vi "PH_Timing.PC link SRDG 645 Channel Infos.vi"(0 "i ref in":refnum<vi>, 1 "data":i8[](array[numeric]), 2 "Service Name":string="N/A", 3 "typeDescriptor":string="D:N", 4 "no link":bool, 5 "error in":errorcluster) -> (14 "i ref out":refnum<vi>, 19 "error out":errorcluster)   [LabVIEW 2014, in "PH_Timing.lvlib"]
doc: "This VI writes the incoming information to own attributes and sets GUI elements."
uses:
  PH_Timing.lvlib
  instr.lib/Stanford Research DG645/Driver/Channel.ctl
  instr.lib/Stanford Research DG645/Stanford Research DG645 - Driver.lvlib
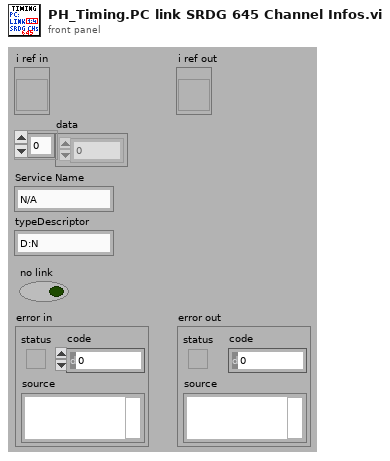
[diagram p1: front panel]
types:
  T1 = typedef "PH_Timing.lvlib/PH_Timing.i attribute.ctl" = cluster{"Sequencer":cluster{"linked?":bool, "Proc State":string, "Ref State":refnum<vi>}, "Gate Generator":cluster{"GD":cluster{"Device Status":T2, "linked?":bool}, "Settings":T3, "GUI Ref":refnum<vi>}, "Interlock Bypass":cluster{"Instancename":string, "Switch linked?":bool, "Device Status":T2, "Ref Status":refnum<vi>}, "Roughtuner":cluster{"Settings":T4, "GUI Ref":refnum<vi>, "GD":cluster{"Device Status":T2, "linked?":bool}}, "0,5Hz Gater":cluster{"Settings":T5, "GUI Ref":refnum<vi>, "GD":cluster{"Device Status":T2, "linked?":bool}}, "Slow Trigger":cluster{"Settings":T6, "GUI Ref":refnum<vi>, "Service ID Delay":i32, "Service ID Ext Trig":i32, "Wanted Settings":T6}, "Timing Mode":cluster{"Mode":T7, "GUI Ref":refnum<vi>, "Service ID T2":i32, "Service ID Mode":i32, "Wanted Mode":T7}, "ns Generator":cluster{"Settings":T8, "ns Generator Settings":refnum<vi>, "GD":cluster{"Device Status":T2, "linked?":bool}}, "Phase FEs":cluster{"Settings":T11, "GUI Ref":refnum<vi>, "Service ID Phase":i32, "Wanted Settings":T11}, "GD GUI Refs":refnum<vi>[], "Heads":T12[], "GUI Ref Delete":refnum<vi>}
  T2 = typedef "PH_StatusHandler.lvlib/PH_StatusHandler.Status.ctl" = i16
  T3 = typedef "PH_Timing.lvlib/PH_Timing.GateGen.ctl" = cluster{"Instance":string, "Channel Gate":i32, "Channel T2":i32, "Width Gate":dbl, "Width T2":dbl, "Delay Gate":dbl, "Delay T2":dbl, "Gate activ":bool, "T2 activ":bool, "System Mode":enum16{"Normal", "Single", "Burst", "Duty Cycle"}}
  T4 = typedef "PH_Timing.lvlib/PH_Timing.Roughtuner.ctl" = cluster{"Instance":string, "Phase PHELIX / UNILAC":cluster{"Channel":u16, "relative to":u16, "Delay [ms]":dbl}, "Pulse Length":cluster{"Channel":u16, "relative to":u16, "Delay [ms]":dbl}, "Trigger":cluster{"externally?":bool, "Rate [Hz]":dbl}}
  T5 = typedef "PH_Timing.lvlib/PH_Timing.0.5HzGater.ctl" = cluster{"Instance":string, "Channel ns FE Delay":i32, "Channel 0.5Hz":i32, "Width ns FE Delay":dbl, "Width 0.5Hz":dbl, "Delay ns FE Delay":dbl, "Delay 0.5Hz":dbl, "ns FE Delay active":bool, "0.5Hz activ":bool, "ns FE Delay inverted":bool, "0.5Hz inverted":bool}
  T6 = typedef "PH_Timing.lvlib/PH_Timing.Slow Trigger Settings.ctl" = cluster{"Delay":dbl, "externally triggered?":bool}
  T7 = typedef "PH_Timing.lvlib/PH_Timing.Timing Mode.ctl" = cluster{"T2":i16, "Modeselector":enum32{"10 Hz", "0.5 Hz", "Shot"}}
  T8 = typedef "PH_Timing.lvlib/PH_Timing.ns Generator.ctl" = cluster{"Instance":string, "Phase fs / ns FE":cluster{"Channel":T9, "Settings":T10}}
  T9 = typedef "Stanford Research DG645 - Driver.lvlib/Channel.ctl" = i32
  T10 = typedef "PH_SRDG645.lvlib/PH_SRDG645.Channel Settings.ctl" = cluster{"Delay [s]":dbl, "relative to":i32}
  T11 = typedef "PH_Timing.lvlib/PH_Timing.Phase FEs.ctl" = cluster{"Phase":dbl}
  T12 = typedef "PH_Timing.lvlib/PH_Timing.PU Data.ctl" = cluster{"linked?":bool, "Data":T13, "GD":cluster{"Device Status":T2, "linked?":bool}, "GUI Ref":refnum<vi>, "PU":T14}
  T13 = typedef "PH_Timing.lvlib/PH_Timing.PU Info.ctl" = cluster{"Act CH?":bool, "GD":string, "CH":i32, "Delay":dbl, "active":bool, "in Use?":bool}
  T14 = typedef "PH_PP_Common.lvlib/PH_PP_Common.PUs.ctl" = enum16{"no Info", "PA-19mm-1", "PA-19mm-2", "PA-45mm-PILC", "PA-45mm-MAIN", "MA-PU-1", "MA-PU-2", "MA-PU-3", "MA-PU-4", "MA-PU-5", "MA-PU-6", "MA-FR", "MA-PILC", "PA-45mm-DP"}
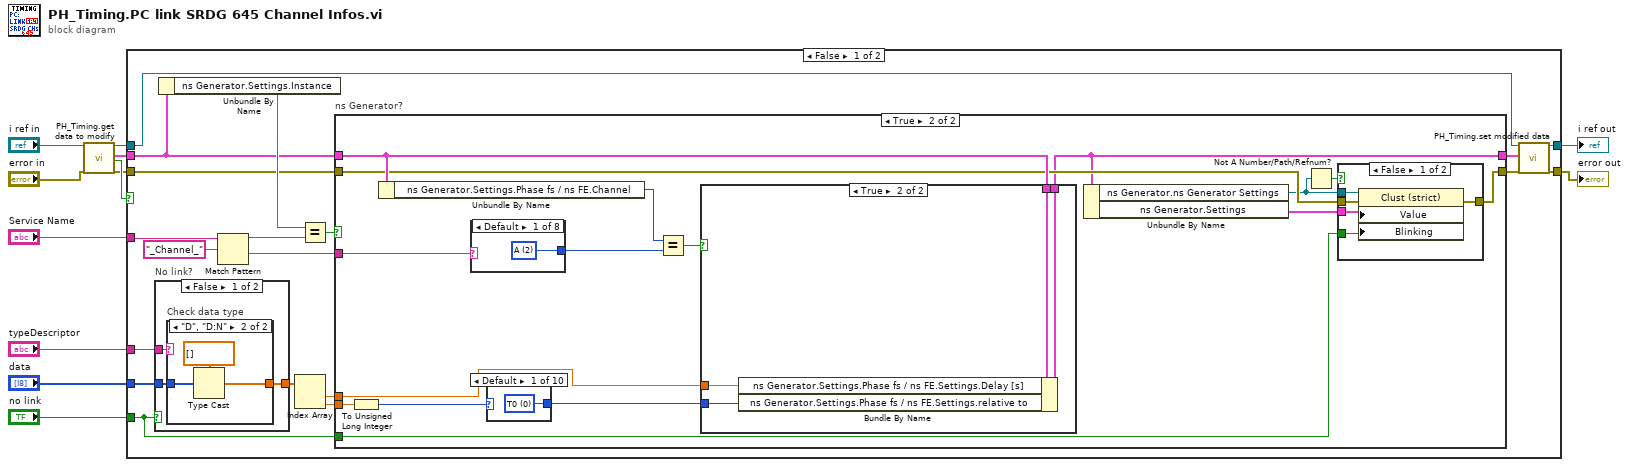
[diagram p0: block diagram]
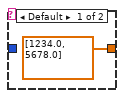
[diagram p2: hidden frame]
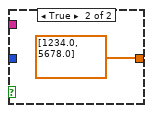
[diagram p3: hidden frame]
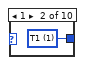
[diagram p5: hidden frame]
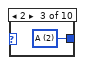
[diagram p6: hidden frame]
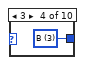
[diagram p7: hidden frame]
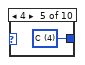
[diagram p8: hidden frame]
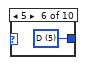
[diagram p9: hidden frame]
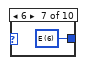
[diagram p10: hidden frame]
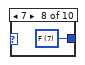
[diagram p11: hidden frame]
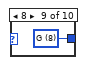
[diagram p12: hidden frame]
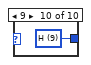
[diagram p13: hidden frame]
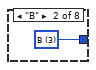
[diagram p15: hidden frame]
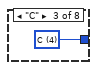
[diagram p16: hidden frame]
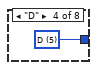
[diagram p17: hidden frame]
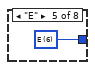
[diagram p18: hidden frame]
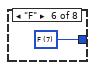
[diagram p19: hidden frame]
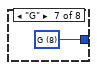
[diagram p20: hidden frame]
diagram:
  n1 = call "PH_Timing.get data to modify.vi"("i ref in"="i ref in", "error in (no error)"="error in") -> ("i ref out"=w4:refnum<vi>, "i attribute"=w9:T1, "timed out"=w10:bool, "error out"=w7:errorcluster)  [unwired: 14 in]
  n2 = case shown="False" w10 {
    tunnel: w4 -> [w13 w88]
    tunnel: [w31 w88] -> w5
    tunnel: w7 -> [w16 w87]
    tunnel: [w30 w87] -> w8
    tunnel: w9 -> [w14 _]
    tunnel: "no link" -> [w20 _]
    tunnel: "Service Name" -> [w29 _]
    tunnel: "data" -> [w26 _]
    tunnel: "typeDescriptor" -> [w25 _]
    frame False {
      n3 = case "No link?" shown="False" w20 {
        tunnel: [w34 dbl[] [1234.0, 5678.0]] -> w24
        tunnel: w26 -> [w33 _]
        tunnel: w25 -> [w32 _]
        frame False {
          n4 = case "Check data type" shown="\"D\", \"D:N\"" w32 {
            tunnel: [dbl[] [1234.0, 5678.0] w37] -> w34
            tunnel: w33 -> [_ w38]
            frame Default {
            }
            frame "D", "D:N" {
              n5 = Type Cast(type=dbl[] [], x=w38) -> (*(type *) &x=w37:dbl[])
            }
          }
        }
        frame True {
        }
      }
      n6 = Unbundle By Name(w14) -> ("ns Generator.Settings.Instance"=w19:string)
      n7 = Match Pattern(string=w29, regular expression="_Channel_") -> (before substring=w18:string, after substring=w15:string)  [unwired: 1 in, 2 out]
      n8 = Index Array(array=w24) -> (element #1=w23:dbl, element #2=w22:dbl)  [unwired: 2 in]
      n9 = Equal?(x=w19, y=w18) -> (x = y?=w17:bool)
      n10 = case "ns Generator?" shown="True" w17 {
        tunnel: w14 -> [w41 w55]
        tunnel: [w41 w51] -> w27
        tunnel: w23 -> [_ w42]
        tunnel: w22 -> [_ w56]
        tunnel: w16 -> [w40 w54]
        tunnel: [w40 w53] -> w21
        tunnel: w20 -> [_ w52]
        tunnel: w15 -> [_ w57]
        frame False {
        }
        frame True {
          n11 = To Unsigned Long Integer(number=w56) -> (unsigned 32bit integer=w44:u32)
          n12 = Unbundle By Name(w55) -> ("ns Generator.Settings.Phase fs / ns FE.Channel"=w47:T9)
          n13 = case shown="Default" w57 {
            tunnel: [w74 w75 w76 w77 w78 w79 w80 w81] -> w46
            frame Default {
              w74 = T9 2 items=["T0", "T1", "A", "B", "C", "D", "E", "F", "G", "H"] ("ns Generator.Settings.Phase fs / ns FE.Channel")
            }
            frame "B" {
              w75 = T9 3 items=["T0", "T1", "A", "B", "C", "D", "E", "F", "G", "H"] ("ns Generator.Settings.Phase fs / ns FE.Channel")
            }
            frame "C" {
              w76 = T9 4 items=["T0", "T1", "A", "B", "C", "D", "E", "F", "G", "H"] ("ns Generator.Settings.Phase fs / ns FE.Channel")
            }
            frame "D" {
              w77 = T9 5 items=["T0", "T1", "A", "B", "C", "D", "E", "F", "G", "H"] ("ns Generator.Settings.Phase fs / ns FE.Channel")
            }
            frame "E" {
              w78 = T9 6 items=["T0", "T1", "A", "B", "C", "D", "E", "F", "G", "H"] ("ns Generator.Settings.Phase fs / ns FE.Channel")
            }
            frame "F" {
              w79 = T9 7 items=["T0", "T1", "A", "B", "C", "D", "E", "F", "G", "H"] ("ns Generator.Settings.Phase fs / ns FE.Channel")
            }
            frame "G" {
              w80 = T9 8 items=["T0", "T1", "A", "B", "C", "D", "E", "F", "G", "H"] ("ns Generator.Settings.Phase fs / ns FE.Channel")
            }
            frame "H" {
              w81 = T9 9 items=["T0", "T1", "A", "B", "C", "D", "E", "F", "G", "H"] ("ns Generator.Settings.Phase fs / ns FE.Channel")
            }
          }
          n14 = case shown="Default" w44 {
            tunnel: [w58 w59 w60 w61 w62 w63 w64 w65 w66 w67] -> w43
            frame Default {
              w58 = T9 0 items=["T0", "T1", "A", "B", "C", "D", "E", "F", "G", "H"] ("ns Generator.Settings.Phase fs / ns FE.Channel")
            }
            frame 1 {
              w59 = T9 1 items=["T0", "T1", "A", "B", "C", "D", "E", "F", "G", "H"] ("ns Generator.Settings.Phase fs / ns FE.Channel")
            }
            frame 2 {
              w60 = T9 2 items=["T0", "T1", "A", "B", "C", "D", "E", "F", "G", "H"] ("ns Generator.Settings.Phase fs / ns FE.Channel")
            }
            frame 3 {
              w61 = T9 3 items=["T0", "T1", "A", "B", "C", "D", "E", "F", "G", "H"] ("ns Generator.Settings.Phase fs / ns FE.Channel")
            }
            frame 4 {
              w62 = T9 4 items=["T0", "T1", "A", "B", "C", "D", "E", "F", "G", "H"] ("ns Generator.Settings.Phase fs / ns FE.Channel")
            }
            frame 5 {
              w63 = T9 5 items=["T0", "T1", "A", "B", "C", "D", "E", "F", "G", "H"] ("ns Generator.Settings.Phase fs / ns FE.Channel")
            }
            frame 6 {
              w64 = T9 6 items=["T0", "T1", "A", "B", "C", "D", "E", "F", "G", "H"] ("ns Generator.Settings.Phase fs / ns FE.Channel")
            }
            frame 7 {
              w65 = T9 7 items=["T0", "T1", "A", "B", "C", "D", "E", "F", "G", "H"] ("ns Generator.Settings.Phase fs / ns FE.Channel")
            }
            frame 8 {
              w66 = T9 8 items=["T0", "T1", "A", "B", "C", "D", "E", "F", "G", "H"] ("ns Generator.Settings.Phase fs / ns FE.Channel")
            }
            frame 9 {
              w67 = T9 9 items=["T0", "T1", "A", "B", "C", "D", "E", "F", "G", "H"] ("ns Generator.Settings.Phase fs / ns FE.Channel")
            }
          }
          n15 = Equal?(x=w47, y=w46) -> (x = y?=w45:bool)
          n16 = case shown="True" w45 {
            tunnel: w42 -> [_ w83]
            tunnel: w43 -> [_ w86]
            tunnel: w55 -> [w82 w85]
            tunnel: [w82 w84] -> w51
            frame False {
            }
            frame True {
              n17 = Bundle By Name(cluster=w85, "ns Generator.Settings.Phase fs / ns FE.Settings.Delay [s]"=w83, "ns Generator.Settings.Phase fs / ns FE.Settings.relative to"=w86) -> (w84:T1)
            }
          }
          n18 = Unbundle By Name(w51) -> ("ns Generator.ns Generator Settings"=w49:refnum<vi>, "ns Generator.Settings"=w48:T8)
          n19 = Not A Number/Path/Refnum?(number/path/refnum=w49) -> (NaN/Path/Refnum?=w50:bool)
          n20 = case shown="False" w50 {
            tunnel: [w72 w73] -> w53
            tunnel: w54 -> [w71 w73]
            tunnel: w52 -> [w70 _]
            tunnel: w49 -> [w69 _]
            tunnel: w48 -> [w68 _]
            frame False {
              n21 = property class="Clust (strict)"(reference=w69, error in=w71, "Value"=w68, "Blinking"=w70) -> (error out=w72:errorcluster)  [unwired: 1 out]
            }
            frame True {
            }
          }
        }
      }
      n22 = call "PH_Timing.set modified data.vi"("i ref in"=w13, "i attribute"=w27, "error in (no error)"=w21) -> ("i ref out"=w31:refnum<vi>, "error out"=w30:errorcluster)  [unwired: 15 in]
    }
    frame True {
    }
  }
  "error out" <- w8
  "i ref out" <- w5
